vi "LWXPS_PositionerMotorOutputOffsetSet.vi"(0 "Primary DAC 1":dbl, 1 "Positioner Name":string, 2 "XPS Reference IN":refnum<k24>, 5 "Primary DAC 2":dbl, 7 "Primary DAC Differential Gain":dbl, 9 "Secondary DAC 1":dbl, 11 "Secondary DAC 2":dbl, 12 "Secondary DAC Differential Gain":dbl, 13 "LabVIEW error IN":errorcluster) -> (4 "XPS Reference OUT":refnum<k24>, 6 "Returned error code":i32, 10 "XPS Error String":string, 15 "LabVIEW error OUT":errorcluster)   [LabVIEW 2014]
uses:
  D:/XPSQ8_LabView_Library/Development/Source/Dll/Newport.XPS.CommandInterface.dll
  Dll/Newport.XPS.CommandInterface.dll
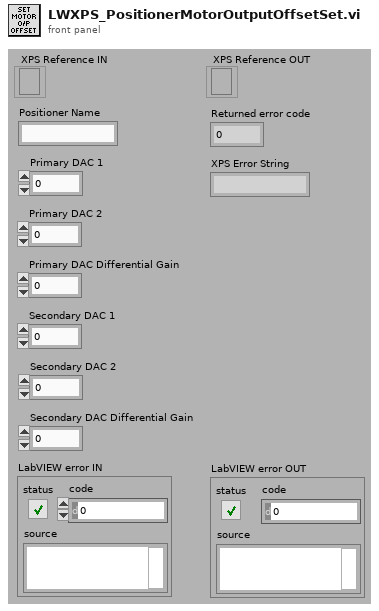
[diagram p1: front panel]
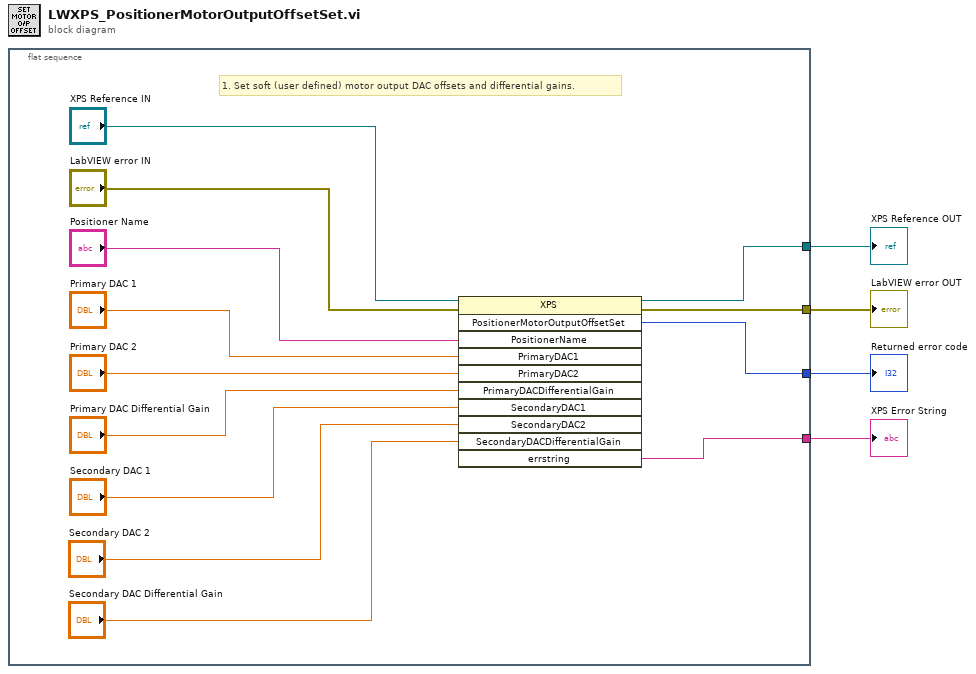
[diagram p0: block diagram]
diagram:
  n1 = flat-sequence {
    tunnel: [w15] -> w4
    tunnel: [w14] -> w3
    tunnel: [w16] -> w2
    tunnel: [w5] -> w1
    frame #0 {
      # "1. Set soft (user defined) motor output DAC offsets and differential gains."
      n2 = invoke class="XPS" method="PositionerMotorOutputOffsetSet"(reference="XPS Reference IN", error in="LabVIEW error IN", "PositionerName"="Positioner Name", "PrimaryDAC1"="Primary DAC 1", "PrimaryDAC2"="Primary DAC 2", "PrimaryDACDifferentialGain"="Primary DAC Differential Gain", "SecondaryDAC1"="Secondary DAC 1", "SecondaryDAC2"="Secondary DAC 2", "SecondaryDACDifferentialGain"="Secondary DAC Differential Gain") -> (reference out=w15:refnum<k24>, error out=w14:errorcluster, "PositionerMotorOutputOffsetSet"=w16:i32, "errstring"=w5:string)  [unwired: 2 in, 7 out]
    }
  }
  "XPS Error String" <- w1
  "XPS Reference OUT" <- w4
  "LabVIEW error OUT" <- w3
  "Returned error code" <- w2
